vi "Draw Circle.vi"(9 "BG Image Property In":T1={"Radius"=[], "Plot Area Bounds"={"Left"=0, "Top"=0, "Right"=0, "Bottom"=0}, "Center position"={"X"=0, "Y"=0}, "Flip?"=FALSE, "Major Gird Color"=10066176, "Minor Gird Color"=5000192}, 11 "Picture In":picture) -> (1 "BG Image Property Out":T1={"Radius"=[], "Plot Area Bounds"={"Left"=0, "Top"=0, "Right"=0, "Bottom"=0}, "Center position"={"X"=0, "Y"=0}, "Flip?"=FALSE, "Major Gird Color"=10066176, "Minor Gird Color"=5000192}, 3 "Picture Out":picture)   [LabVIEW 2017, in "2D Compass.lvclass"]
uses:
  <vilib>/Math Plots/2D Math Plots/2D Compass/2D Compass/2D Compass.lvclass
  <vilib>/Math Plots/2D Math Plots/2D Compass/2D Compass/Typedef/BG Image Property.ctl
  <vilib>/Utility/miscctls.llb/LVRectTypeDef.ctl
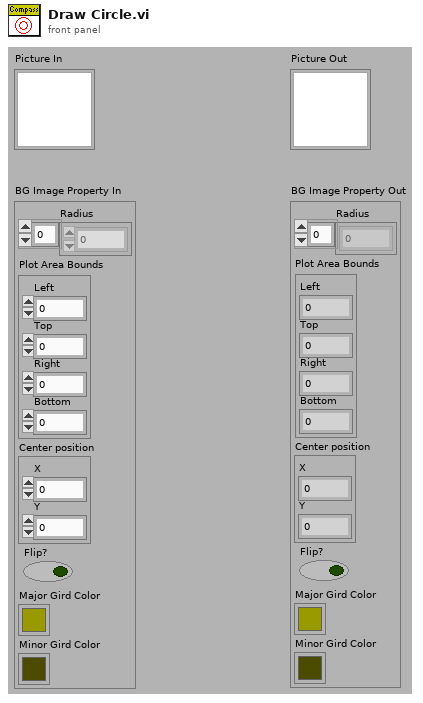
[diagram p1: front panel]
types:
  T1 = typedef "2D Compass.lvclass/BG Image Property.ctl" = cluster{"Radius":i16[], "Plot Area Bounds":T2, "Center position":cluster{"X":i16, "Y":i16}, "Flip?":bool, "Major Gird Color":u32, "Minor Gird Color":u32}
  T2 = typedef "LVRectTypeDef.ctl" = cluster{"Left":i16, "Top":i16, "Right":i16, "Bottom":i16}
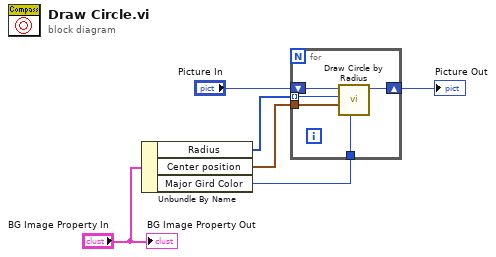
[diagram p0: block diagram]
diagram:
  n1 = Unbundle By Name("BG Image Property In") -> ("Radius"=w2:i16[], "Center position"=w6:cluster{"X":i16, "Y":i16}, "Major Gird Color"=w5:u32)
  n2 = for {
    shift-right: [w10] -> w3
    shift-left: "Picture In" -> [w11]
    tunnel: w6 -> [w9]
    tunnel: w5 -> [w8]
    tunnel: w2 -> [w7] mode=indexing
    n3 = call <vilib>:"Draw Circle by Radius.vi"("color(black)"=w8, "pixel center"=w9, "radius"=w7, "picture"=w11) -> ("new picture"=w10:picture)  [unwired: 4 in, 3 out]
  }
  "Picture Out" <- w3
  "BG Image Property Out" <- "BG Image Property In"
